vi "RT Main v0.91.vi"() -> ()   [LabVIEW 2017]
doc: "Changelog:\n\nv0.9:\n- Autocycle"
uses:
  Controls/Auto Delays.ctl
  support/Controls/All Inputs.ctl
  support/Controls/Index Details.ctl
  support/Controls/Auto Stats.ctl
  Controls/Auto Times.ctl
  Global Variables/RT GV.vi
  support/Message Queue/Enqueue Message (Single).vi
  Global Variables/FPGA GV.vi
  <vilib>/Utility/error.llb/Error Cluster From Error Code.vi
  <vilib>/rvi/errors/niLvFpgaAdjustHostInterfaceError.vi
  Global Variables/Network Globals.vi
  <vilib>/FPGAPlugInAG/Dynamic/niLvFpga_Close_Dynamic.vi
  <vilib>/rvi/interface/nirviReadWriteControl/nirviReadWriteControl.xnode
  Controls/FPGA Ref.ctl
  <vilib>/rvi/interface/nirviCloseFPGA/nirviCloseFPGA.xnode
  support/Message Queue/Message Queue.lvlib
  NiFpgaLv.dll
  <vilib>/rvi/interface/Simulation/niFpgaSimulationCallBeginRW.vi
panel:
  in  "Auto Para":T1={"Agitator Delays"=[700, 250], "TF Delays"=[700, 800, 2], "Insertion Delays"=[100, 500], "Cutting Delays"=[300, 300, 100], "PF Delays"=[250, 30000], "Measur. Delays"=[500.0, 188.9, 1.0], "Reject Delays"=[500], "BF Delays"=[1000, 1000]}
  in  "Counts in":cluster{"OutputCount":u32, "RejectCount":u32}
  in  "Stop Button 4":bool
  out "error out":errorcluster
  out "Wrong Message":string
  in  "Stop Button":bool
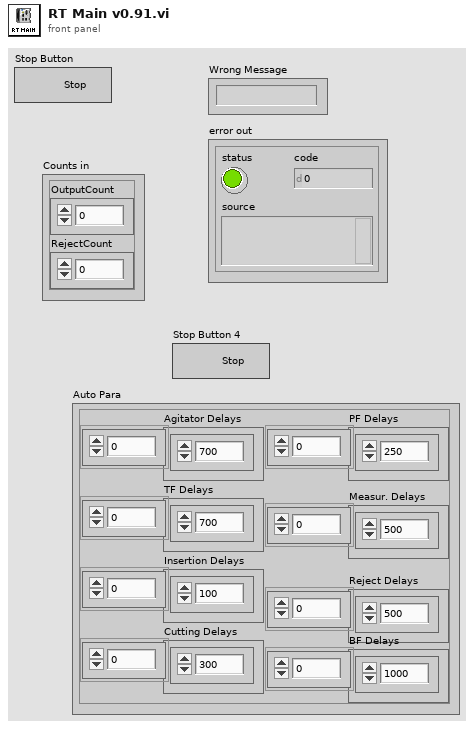
[diagram p1: front panel]
types:
  T1 = typedef "Auto Delays.ctl" = cluster{"Agitator Delays":u32[], "TF Delays":u32[], "Insertion Delays":u32[], "Cutting Delays":u32[], "PF Delays":u32[], "Measur. Delays":dbl[], "Reject Delays":u32[], "BF Delays":u32[]}
  T2 = typedef "FPGA Ref.ctl" = refnum<k20>
  T3 = cluster{"TL_Red":bool, "TL_Orange":bool, "TL_Green":bool, "TL_Buzzer":bool, "SOL_Index_Rotary_CW":bool, "SOL_Index_CNVR_Rotary_CCW":bool, "SOL_Index_CNVR_Stopper_Rear":bool, "SOL_Index_CNVR_Output _Separator _Rear":bool, "Bowl  Feeder_ ON":bool, "Pump_CNVR_Motor _ON":bool, "SOL_Gating_CYL_Rear":bool, "SOL_Tube_Feed_Agitatator":bool, "SOL_Tube_Feed_Gating_CYL":bool, "SOL_Insertion _CYL":bool, "SOL_Insertion_Clamp_CYL":bool, "SOL_Cutting_CYL":bool, "SOL_Cutting_Clamp_CYL":bool, "SOL_Insertion_Air_Nozzle":bool, "SOL_Measurement_CYL":bool, "SOL_Measure_Clamp_CYL":bool, "SOL_Rejection CYL_1":bool, "SOL_Rejection CYL_2":bool, "SOL_Rejection CYL_3":bool, "SOL_Rejection CYL_4":bool, "DO1.24":bool, "DO1.25":bool, "DO1.26":bool, "DO1.27":bool, "DO1.28":bool, "DO1.29":bool, "DO1.30":bool, "DO1.31":bool}
  T4 = typedef "All Inputs.ctl" = cluster{"DI 1":cluster{"Machine_ON":bool, "E_stop ":bool, "SW_Pressure":bool, "SW_Start ":bool, "SW_Reset":bool, "SW_Stop":bool, "SW_Door":bool, "RS_Index_Rotary_CW":bool, "RS_Index_Rotary_CCW":bool, "RS_Index_Stopper _Rear":bool, "RS_Index_Output_Separator_Rear":bool, "PES_Index_Pallet_Sensor":bool, "PES_Index_Output_Part Sensor":bool, "ICS_BF_Low_Level_1":bool, "ICS_BF_Low_Level_2":bool, "ICS_BF_Pump_CNVR_Full_1":bool, "ICS_BF_Pump_CNVR_Full_2":bool, "ICS_BF_Pump_CNVR_Full_3":bool, "ICS_BF_Pump_CNVR_Full_4":bool, "PES_PC_Pump Presence_1":bool, "PES_PC_Pump Presence_2":bool, "PES_PC_Pump Presence_3":bool, "PES_PC_Pump Presence_4":bool, "RS_PC_Gating_Front":bool, "PES_Pump_Interference":bool, "PES_TF_Low_Level":bool, "PES_Tube Presence_1":bool, "PES_Tube Presence_2":bool, "PES_Tube Presence_3":bool, "PES_Tube Presence_4":bool, "DI1.30":bool, "DI1.31":bool}, "DI 2":cluster{"RS_Agitatator_1_Rear ":bool, "RS_Agitatator_2_Rear ":bool, "RS_TF_Gating CYL_Rear":bool, "RS_Insertion_1_Rear":bool, "RS_Insertion_1_Front":bool, "RS_Insertion _2_Rear":bool, "RS_Insertion _2_Front":bool, "RS_Insertion _3_Rear":bool, "RS_Insertion _3_Front":bool, "RS_Insertion _4_Rear":bool, "RS_Insertion _4_Front":bool, "RS_Insertion_Clamp_Rear":bool, "RS_Cutting_Rear":bool, "RS_Cutting_Clamp _Rear":bool, "RS_Measurement_1_Rear":bool, "RS_Measurement_2_Rear":bool, "RS_Measurement_3_Rear":bool, "RS_Measurement_4_Rear":bool, "RS_Measure_Clamp_Rear":bool, "RS_Rejection_1_Rear":bool, "RS_Rejection_2_Rear":bool, "RS_Rejection_3_Rear":bool, "RS_Rejection_4_Rear":bool, "DI2.23":bool, "DI2.24":bool, "DI2.25":bool, "DI2.26":bool, "DI2.27":bool, "DI2.28":bool, "DI2.29":bool, "DI2.30":bool, "DI2.31":bool}, "IAS 1":dbl, "IAS 2":dbl, "IAS 3":dbl, "IAS 4":dbl, "DO 1":cluster{"TL_Red":bool, "TL_Orange":bool, "TL_Green":bool, "TL_Buzzer":bool, "SOL_Index_Rotary_CW":bool, "SOL_Index_CNVR_Rotary_CCW":bool, "SOL_Index_CNVR_Stopper_Rear":bool, "SOL_Index_CNVR_Output _Separator _Rear":bool, "Bowl  Feeder_ ON 1":bool, "Pump_CNVR_Motor _ON":bool, "SOL_PC_Gating_CYL_Rear":bool, "SOL_Tube_Feed_Agitatator":bool, "SOL_Tube_Feed_Gating_CYL":bool, "SOL_Insertion _CYL":bool, "SOL_Insertion_Clamp_CYL":bool, "SOL_Cutting_CYL":bool, "SOL_Cutting_Clamp_CYL":bool, "SOL_Insertion_Air_Nozzle":bool, "SOL_Measurement_CYL":bool, "DO1.19":bool, "SOL_Rejection CYL_1":bool, "SOL_Rejection CYL_2":bool, "SOL_Rejection CYL_3":bool, "SOL_Rejection CYL_4":bool, "Bowl  Feeder_ ON 2":bool, "SOL_BF_BlowerON":bool, "SOL_BF1_Track1":bool, "SOL_BF1_Track2":bool, "SOL_BF2_Track1":bool, "SOL_BF2_Track2":bool, "DO1.30":bool, "DO1.31":bool}}
  T5 = typedef "Index Details.ctl" = cluster{"Time (ms)":u32, "Waveform Graph":i16[]}
  T6 = cluster{T1, "Reject Pallets":cluster{"Reject 1":bool, "Reject 2":bool, "Reject 3":bool, "Reject 4":bool}}
  T7 = typedef "Auto Stats.ctl" = cluster{"Time":timestamp, "OEE":cluster{"AVL":dbl, "PRF":dbl, "QUA":dbl, "OEE":dbl}, "Auto Times":T8, "Counts out":cluster{"OutputCount":u32, "RejectCount":u32}, "Measurements":cluster{"1":dbl, "2":dbl, "3":dbl, "4":dbl}, "Outputs":cluster{"OutputCount":u32, "Numeric Control":u32}}
  T8 = typedef "Auto Times.ctl" = cluster{"Index Time":u32, "TF Time":u32, "Insertion Time":u32, "Cutting Time":u32, "PF Time":u32, "Meas. Time":u32, "Reject Time":u32}
  T9 = cluster{string, dbl, "Counts in":cluster{"OutputCount":u32, "RejectCount":u32}, "Auto Para":T1}
  T10 = cluster{"TL_Red":bool, "TL_Orange":bool, "TL_Green":bool, "TL_Buzzer":bool, "SOL_Index_Rotary_CW":bool, "SOL_Index_CNVR_Rotary_CCW":bool, "SOL_Index_CNVR_Stopper_Rear":bool, "SOL_Index_CNVR_Output _Separator _Rear":bool, "Bowl Feeder_ ON1":bool, "Pump_CNVR_Motor _ON":bool, "SOL_PC_Gating_CYL_Rear":bool, "SOL_Tube_Feed_Agitatator":bool, "SOL_Tube_Feed_Gating_CYL":bool, "SOL_Insertion _CYL":bool, "SOL_Insertion_Clamp_CYL":bool, "SOL_Cutting_CYL":bool, "SOL_Cutting_Clamp_CYL":bool, "SOL_Insertion_Air_Nozzle":bool, "SOL_Measurement_CYL":bool, "DO1.19":bool, "SOL_Rejection CYL_1":bool, "SOL_Rejection CYL_2":bool, "SOL_Rejection CYL_3":bool, "SOL_Rejection CYL_4":bool, "Bowl Feeder_ON2":bool, "SOL_BF_BlowerON":bool, "SOL_BF1_Track1":bool, "SOL_BF1_Track2":bool, "SOL_BF2_Track1":bool, "SOL_BF2_Track2":bool, "DO1.30":bool, "DO1.31":bool}
  T11 = cluster{"Machine_ON":bool, "E_stop ":bool, "SW_Pressure":bool, "SW_Start ":bool, "SW_Reset":bool, "SW_Stop":bool, "SW_Door":bool, "RS_Index_Rotary_CW":bool, "RS_Index_Rotary_CCW":bool, "RS_Index_Stopper _Rear":bool, "RS_Index_Output_Separator_Rear":bool, "PES_Index_Pallet_Sensor":bool, "PES_Index_Output_Part Sensor":bool, "ICS_BF_Low_Level_1":bool, "ICS_BF_Low_Level_2":bool, "ICS_BF_Pump_CNVR_Full_1":bool, "ICS_BF_Pump_CNVR_Full_2":bool, "ICS_BF_Pump_CNVR_Full_3":bool, "ICS_BF_Pump_CNVR_Full_4":bool, "PES_PC_Pump Presence_1":bool, "PES_PC_Pump Presence_2":bool, "PES_PC_Pump Presence_3":bool, "PES_PC_Pump Presence_4":bool, "RS_PC_Gating_Front":bool, "PES_Pump_Interference":bool, "PES_TF_Low_Level":bool, "PES_Tube Presence_1":bool, "PES_Tube Presence_2":bool, "PES_Tube Presence_3":bool, "PES_Tube Presence_4":bool, "DI1.30":bool, "DI1.31":bool}
  T12 = cluster{"RS_Agitatator_1_Rear ":bool, "RS_Agitatator_2_Rear ":bool, "RS_TF_Gating CYL_Rear":bool, "RS_Insertion_1_Rear":bool, "RS_Insertion_1_Front":bool, "RS_Insertion _2_Rear":bool, "RS_Insertion _2_Front":bool, "RS_Insertion _3_Rear":bool, "RS_Insertion _3_Front":bool, "RS_Insertion _4_Rear":bool, "RS_Insertion _4_Front":bool, "RS_Insertion_Clamp_Rear":bool, "RS_Cutting_Rear":bool, "RS_Cutting_Clamp _Rear":bool, "RS_Measurement_1_Rear":bool, "RS_Measurement_2_Rear":bool, "RS_Measurement_3_Rear":bool, "RS_Measurement_4_Rear":bool, "DI2.18":bool, "RS_Rejection_1_Rear":bool, "RS_Rejection_2_Rear":bool, "RS_Rejection_3_Rear":bool, "RS_Rejection_4_Rear":bool, "DI2.23":bool, "DI2.24":bool, "DI2.25":bool, "DI2.26":bool, "DI2.27":bool, "DI2.28":bool, "DI2.29":bool, "DI2.30":bool, "DI2.31":bool}
  T13 = cluster{"Array":string[][], "Machine Status":string}
  T14 = cluster{"Measurements":cluster{"1":dbl, "2":dbl, "3":dbl, "4":dbl}, "Reject Pallets":cluster{"Reject 1":bool, "Reject 2":bool, "Reject 3":bool, "Reject 4":bool}}
  T15 = cluster{"Auto Times":T8, "Results":cluster{"Measurements":cluster{"1":dbl, "2":dbl, "3":dbl, "4":dbl}, "Reject Pallets":cluster{"Reject 1":bool, "Reject 2":bool, "Reject 3":bool, "Reject 4":bool}}, "OutputCount":u32, "error out":errorcluster}
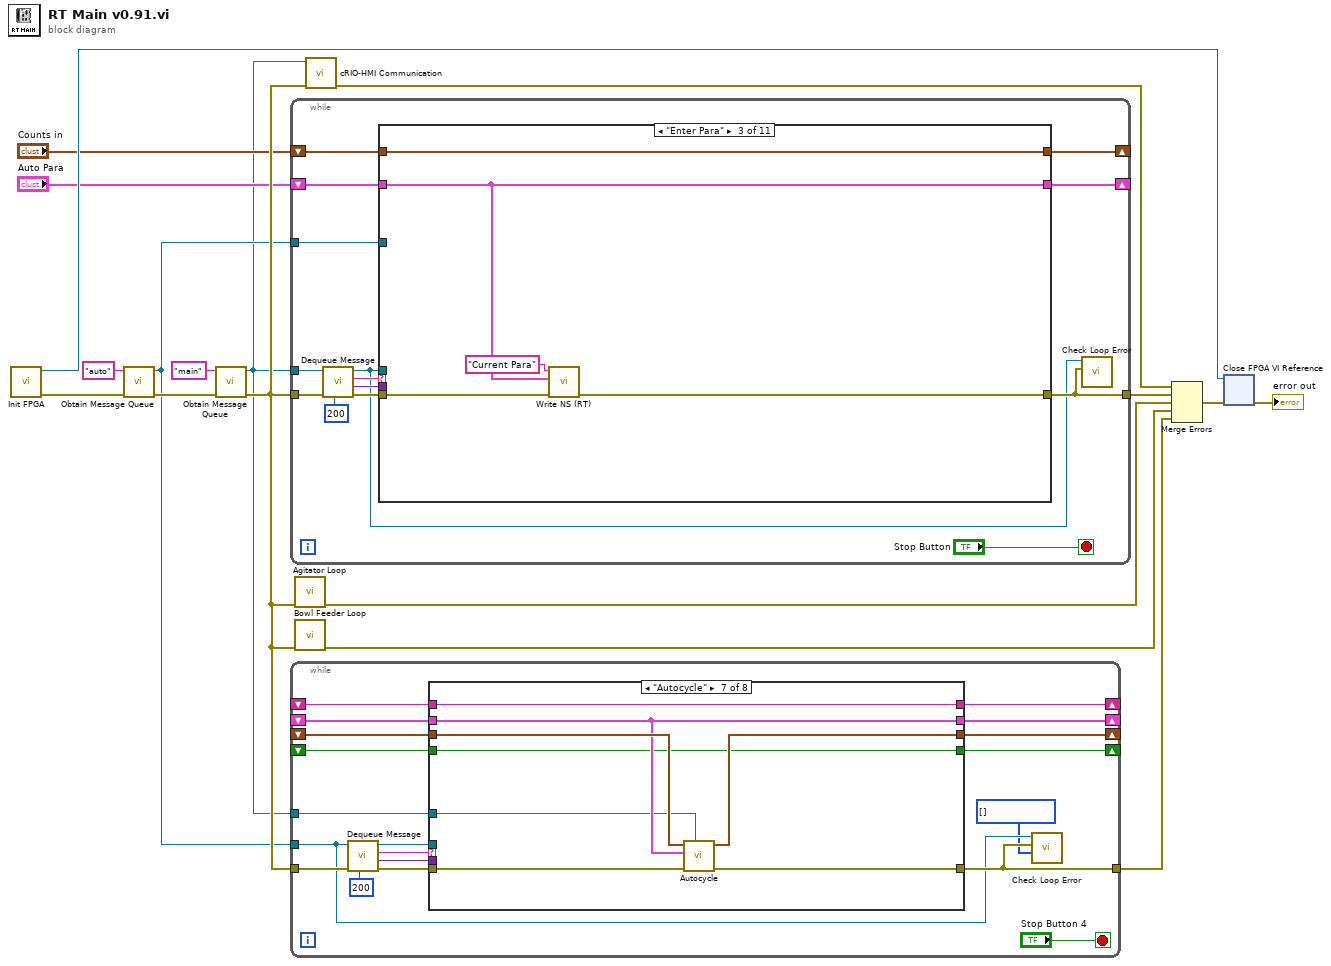
[diagram p0: block diagram]
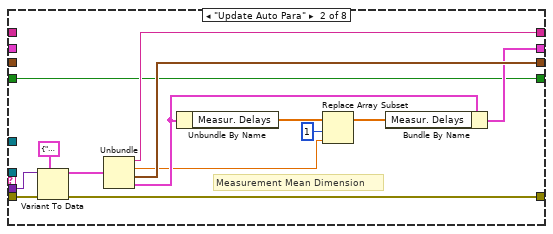
[diagram p3: hidden frame]
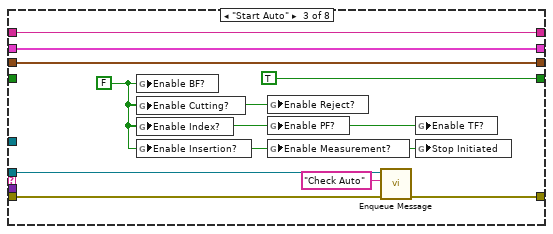
[diagram p4: hidden frame]
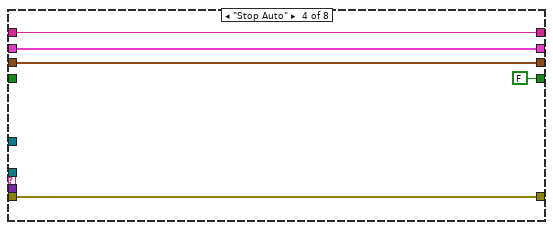
[diagram p5: hidden frame]
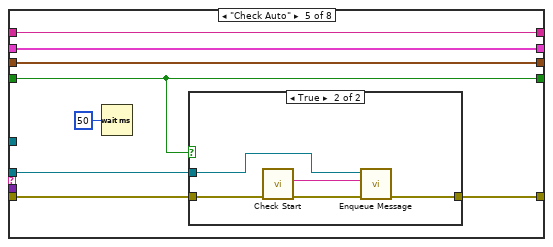
[diagram p6: hidden frame]
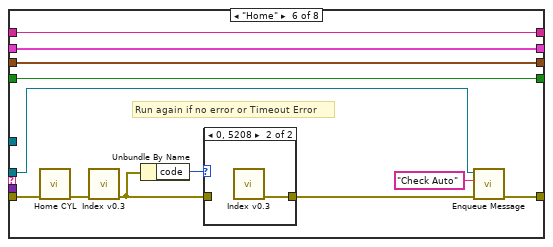
[diagram p8: hidden frame]
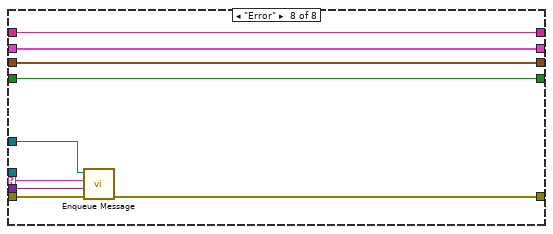
[diagram p10: hidden frame]
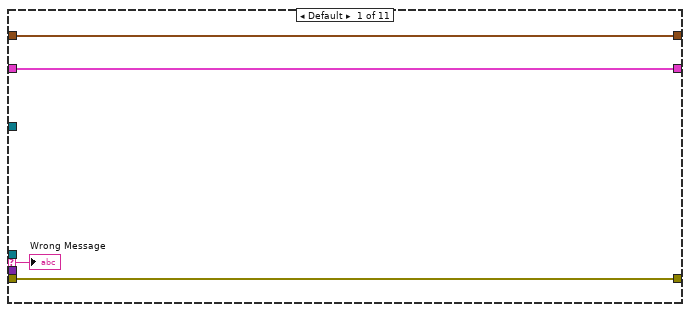
[diagram p11: hidden frame]
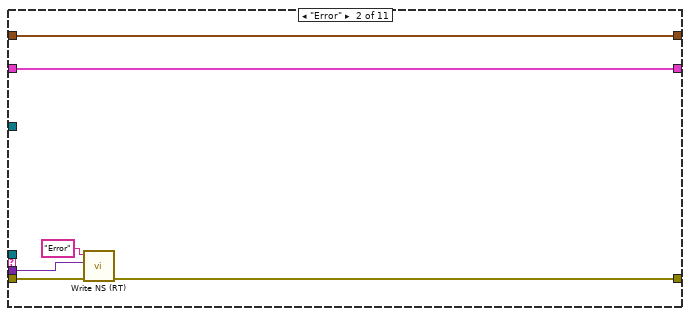
[diagram p12: hidden frame]
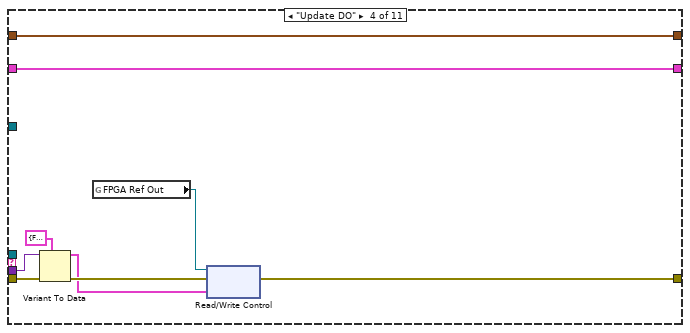
[diagram p13: hidden frame]
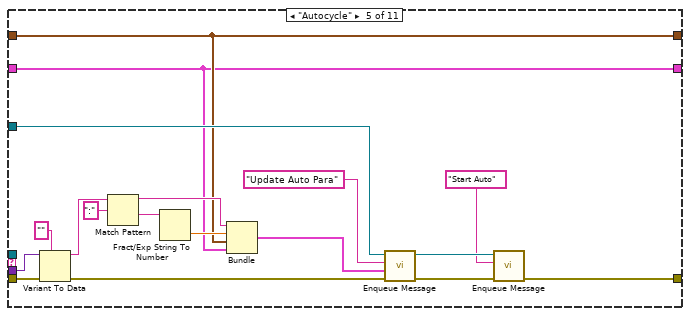
[diagram p14: hidden frame]
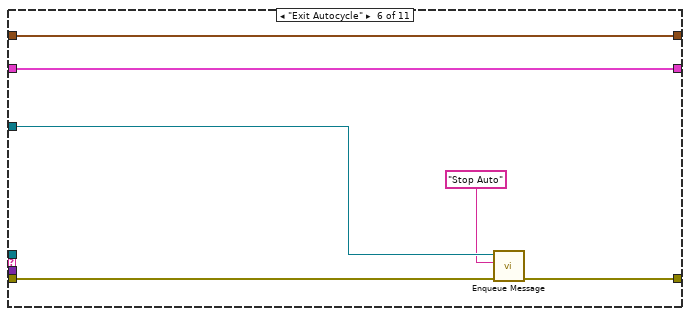
[diagram p15: hidden frame]
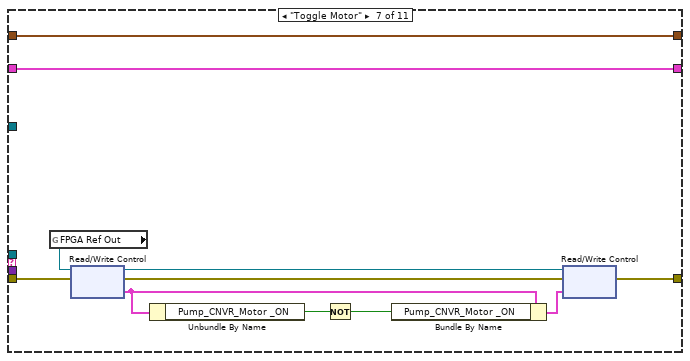
[diagram p16: hidden frame]
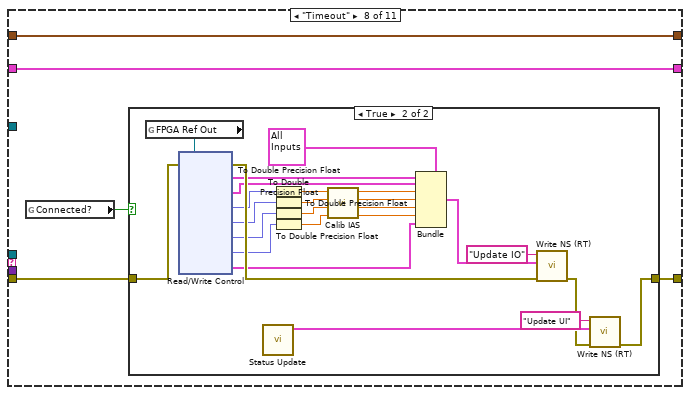
[diagram p17: hidden frame]
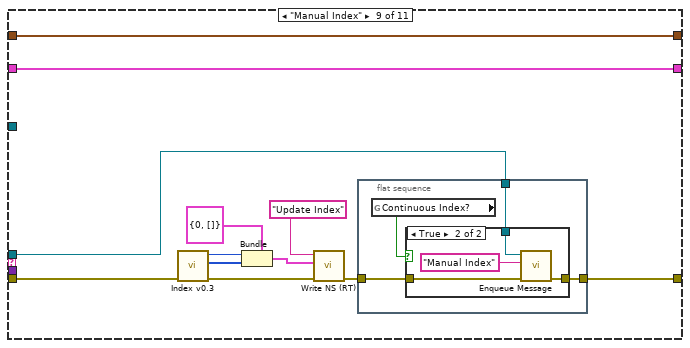
[diagram p19: hidden frame]
diagram:
  n1 = call "Init FPGA.vi"() -> ("error out"=w6:errorcluster, "FPGA Ref Out"=w11:T2)  [unwired: 10 in]
  n2 = call "Obtain Message Queue.vi"("error in (no error)"=w6, "name"="auto") -> ("error out"=w5:errorcluster, "Message Queue"=w2:refnum<queue>)  [unwired: 8 in]
  n3 = call "Obtain Message Queue.vi"("error in (no error)"=w5, "name"="main") -> ("error out"=w10:errorcluster, "Message Queue"=w1:refnum<queue>)  [unwired: 8 in]
  n4 = while {
    tunnel: w10 -> [w30]
    tunnel: w1 -> [w29]
    tunnel: [w25] -> w17
    tunnel: w2 -> [w22]
    shift-right: [w19] -> _
    shift-left: "Auto Para" -> [w20]
    shift-right: [w18] -> _
    shift-left: "Counts in" -> [w21]
    stop <- "Stop Button" stop-if-true
    n5 = call "Dequeue Message.vi"("timeout"=200, "error in (no error)"=w30, "Message Queue"=w29) -> ("error out"=w28:errorcluster, "Message Data"=w26:variant, "Message"=w27:string, "dup Message Queue"=w24:refnum<queue>)  [unwired: 5 in]
    n6 = case shown="\"Enter Para\"" w27 {
      selector: w27 -> [w35 _ _ _ _ _ _ _ _ _ _]
      tunnel: w28 -> [w34 w39 w46 w55 w73 w79 w89 w94 w133 w160 w170]
      tunnel: w24 -> [_ _ _ _ _ _ _ _ w125 _ _]
      tunnel: w26 -> [_ w37 _ w54 w72 _ _ _ _ w159 w169]
      tunnel: [w34 w38 w45 w50 w58 w75 w87 w95 w126 w155 w166] -> w25
      tunnel: w22 -> [_ _ _ _ w65 w78 _ _ _ _ _]
      tunnel: w21 -> [w33 w41 w43 w48 w62 w77 w81 w92 w122 w146 w165]
      tunnel: w20 -> [w32 w40 w42 w47 w61 w76 w80 w91 w123 w145 w164]
      tunnel: [w32 w40 w42 w47 w61 w76 w80 w91 w123 w145 w164] -> w19
      tunnel: [w33 w41 w43 w48 w62 w77 w81 w92 w122 w146 w165] -> w18
      frame Default {
        "Wrong Message" <- w35
      }
      frame "Error" {
        n7 = call "Write NS (RT).vi"("error in (no error)"=w39, "Message Data"=w37, "Message"="Error") -> ("error out"=w38:errorcluster)  [unwired: 8 in]
      }
      frame "Enter Para" {
        n8 = call "Write NS (RT).vi"("error in (no error)"=w46, "Message Data"=w42, "Message"="Current Para") -> ("error out"=w45:errorcluster)  [unwired: 8 in]
      }
      frame "Update DO" {
        n9 = Variant To Data(error in=w55, type=T3 {"TL_Red"=FALSE, "TL_Orange"=FALSE, "TL_Green"=FALSE, "TL_Buzzer"=FALSE, "SOL_Index_Rotary_CW"=FALSE, "SOL_Index_CNVR_Rotary_CCW"=FALSE, "SOL_Index_CNVR_Stopper_Rear"=FALSE, "SOL_Index_CNVR_Output _Separator _Rear"=FALSE, "Bowl  Feeder_ ON"=FALSE, "Pump_CNVR_Motor _ON"=FALSE, "SOL_Gating_CYL_Rear"=FALSE, "SOL_Tube_Feed_Agitatator"=FALSE, "SOL_Tube_Feed_Gating_CYL"=FALSE, "SOL_Insertion _CYL"=FALSE, "SOL_Insertion_Clamp_CYL"=FALSE, "SOL_Cutting_CYL"=FALSE, "SOL_Cutting_Clamp_CYL"=FALSE, "SOL_Insertion_Air_Nozzle"=FALSE, "SOL_Measurement_CYL"=FALSE, "SOL_Measure_Clamp_CYL"=FALSE, "SOL_Rejection CYL_1"=FALSE, "SOL_Rejection CYL_2"=FALSE, "SOL_Rejection CYL_3"=FALSE, "SOL_Rejection CYL_4"=FALSE, "DO1.24"=FALSE, "DO1.25"=FALSE, "DO1.26"=FALSE, "DO1.27"=FALSE, "DO1.28"=FALSE, "DO1.29"=FALSE, "DO1.30"=FALSE, "DO1.31"=FALSE} ("DO 1"), Variant=w54) -> (data=w49:T3, error out=w51:errorcluster)
        n10 = global read "FPGA GV.vi" "FPGA Ref Out"() -> (w52:T2)
        n11 = xnode "Read/Write Control"("FPGA VI Reference In"=w52, "error in"=w51, "DO 1"=w49) -> ("error out"=w50:errorcluster)  [unwired: 1 out]
      }
      frame "Autocycle" {
        n12 = Variant To Data(error in=w73, type="", Variant=w72) -> (data=w68:string, error out=w66:errorcluster)
        n13 = Match Pattern(string=w68, regular expression=":") -> (before substring=w64:string, after substring=w69:string)  [unwired: 1 in, 2 out]
        n14 = Fract/Exp String To Number(string=w69) -> (number=w63:dbl)  [unwired: 3 in, 1 out]
        n15 = Bundle(w64, w63, "Counts in"=w62, "Auto Para"=w61) -> (w60:T9)  [unwired: 1 in]
        n16 = call-poly "Enqueue Message.vi"("error in (no error)"=w66, "Message Data"=w60, "Message"="Update Auto Para", "Message Queue"=w65) -> ("error out"=w59:errorcluster, "dup Message Queue"=w57:refnum<queue>)  [unwired: 6 in]
        n17 = call-poly "Enqueue Message.vi"("error in (no error)"=w59, "Message"="Start Auto", "Message Queue"=w57) -> ("error out"=w58:errorcluster)  [unwired: 7 in, 1 out]
      }
      frame "Exit Autocycle" {
        n18 = call-poly "Enqueue Message.vi"("error in (no error)"=w79, "Message"="Stop Auto", "Message Queue"=w78) -> ("error out"=w75:errorcluster)  [unwired: 7 in, 1 out]
      }
      frame "Toggle Motor" {
        n19 = global read "FPGA GV.vi" "FPGA Ref Out"() -> (w90:T2)
        n20 = xnode "Read/Write Control"("FPGA VI Reference In"=w90, "error in"=w89) -> ("FPGA VI Reference Out"=w86:T2, "error out"=w88:errorcluster, "DO 1"=w84:T10)
        n21 = Unbundle By Name(w84) -> ("Pump_CNVR_Motor _ON"=w85:bool)
        n22 = Not(x=w85) -> (.not. x?=w82:bool)
        n23 = Bundle By Name(cluster=w84, "Pump_CNVR_Motor _ON"=w82) -> (w83:T10)
        n24 = xnode "Read/Write Control"("FPGA VI Reference In"=w86, "error in"=w88, "DO 1"=w83) -> ("error out"=w87:errorcluster)  [unwired: 1 out]
      }
      frame "Timeout" {
        n25 = global read "Network Globals.vi" "Connected?"() -> (w93:bool)
        n26 = case shown="True" w93 {
          tunnel: [w96 w98] -> w95
          tunnel: w94 -> [w96 w120]
          frame False {
          }
          frame True {
            n27 = global read "FPGA GV.vi" "FPGA Ref Out"() -> (w97:T2)
            n28 = xnode "Read/Write Control"("FPGA VI Reference In"=w97, "error in"=w120) -> ("error out"=w119:errorcluster, "DI 1"=w118:T11, "DI 2"=w117:T12, "AI0"=w116:fxp<+/-,27,6>, "AI1"=w115:fxp<+/-,27,6>, "AI2"=w114:fxp<+/-,27,6>, "AI3"=w113:fxp<+/-,27,6>, "DO 1"=w110:T10)  [unwired: 1 out]
            n29 = call "Status Update.vi"() -> ("Status Cluster"=w100:T13)  [unwired: 11 in]
            n30 = To Double Precision Float(number=w116) -> (double precision float=w103:dbl)
            n31 = To Double Precision Float(number=w115) -> (double precision float=w105:dbl)
            n32 = To Double Precision Float(number=w114) -> (double precision float=w107:dbl)
            n33 = To Double Precision Float(number=w113) -> (double precision float=w109:dbl)
            n34 = call "Calib IAS.vi"("x 4"=w109, "x 3"=w107, "x 2"=w105, "x"=w103) -> ("y 4"=w108:dbl, "y 3"=w106:dbl, "y 2"=w104:dbl, "y 1"=w102:dbl)  [unwired: 4 in]
            n35 = Bundle(cluster=T4 {"DI 1"={"Machine_ON"=FALSE, "E_stop "=FALSE, "SW_Pressure"=FALSE, "SW_Start "=FALSE, "SW_Reset"=FALSE, "SW_Stop"=FALSE, "SW_Door"=FALSE, "RS_Index_Rotary_CW"=FALSE, "RS_Index_Rotary_CCW"=FALSE, "RS_Index_Stopper _Rear"=FALSE, "RS_Index_Output_Separator_Rear"=FALSE, "PES_Index_Pallet_Sensor"=FALSE, "PES_Index_Output_Part Sensor"=FALSE, "ICS_BF_Low_Level_1"=FALSE, "ICS_BF_Low_Level_2"=FALSE, "ICS_BF_Pump_CNVR_Full_1"=FALSE, "ICS_BF_Pump_CNVR_Full_2"=FALSE, "ICS_BF_Pump_CNVR_Full_3"=FALSE, "ICS_BF_Pump_CNVR_Full_4"=FALSE, "PES_PC_Pump Presence_1"=FALSE, "PES_PC_Pump Presence_2"=FALSE, "PES_PC_Pump Presence_3"=FALSE, "PES_PC_Pump Presence_4"=FALSE, "RS_PC_Gating_Front"=FALSE, "PES_Pump_Interference"=FALSE, "PES_TF_Low_Level"=FALSE, "PES_Tube Presence_1"=FALSE, "PES_Tube Presence_2"=FALSE, "PES_Tube Presence_3"=FALSE, "PES_Tube Presence_4"=FALSE, "DI1.30"=FALSE, "DI1.31"=FALSE}, "DI 2"={"RS_Agitatator_1_Rear "=FALSE, "RS_Agitatator_2_Rear "=FALSE, "RS_TF_Gating CYL_Rear"=FALSE, "RS_Insertion_1_Rear"=FALSE, "RS_Insertion_1_Front"=FALSE, "RS_Insertion _2_Rear"=FALSE, "RS_Insertion _2_Front"=FALSE, "RS_Insertion _3_Rear"=FALSE, "RS_Insertion _3_Front"=FALSE, "RS_Insertion _4_Rear"=FALSE, "RS_Insertion _4_Front"=FALSE, "RS_Insertion_Clamp_Rear"=FALSE, "RS_Cutting_Rear"=FALSE, "RS_Cutting_Clamp _Rear"=FALSE, "RS_Measurement_1_Rear"=FALSE, "RS_Measurement_2_Rear"=FALSE, "RS_Measurement_3_Rear"=FALSE, "RS_Measurement_4_Rear"=FALSE, "RS_Measure_Clamp_Rear"=FALSE, "RS_Rejection_1_Rear"=FALSE, "RS_Rejection_2_Rear"=FALSE, "RS_Rejection_3_Rear"=FALSE, "RS_Rejection_4_Rear"=FALSE, "DI2.23"=FALSE, "DI2.24"=FALSE, "DI2.25"=FALSE, "DI2.26"=FALSE, "DI2.27"=FALSE, "DI2.28"=FALSE, "DI2.29"=FALSE, "DI2.30"=FALSE, "DI2.31"=FALSE}, "IAS 1"=0.0, "IAS 2"=0.0, "IAS 3"=0.0, "IAS 4"=0.0, "DO 1"={"TL_Red"=FALSE, "TL_Orange"=FALSE, "TL_Green"=FALSE, "TL_Buzzer"=FALSE, "SOL_Index_Rotary_CW"=FALSE, "SOL_Index_CNVR_Rotary_CCW"=FALSE, "SOL_Index_CNVR_Stopper_Rear"=FALSE, "SOL_Index_CNVR_Output _Separator _Rear"=FALSE, "Bowl  Feeder_ ON 1"=FALSE, "Pump_CNVR_Motor _ON"=FALSE, "SOL_PC_Gating_CYL_Rear"=FALSE, "SOL_Tube_Feed_Agitatator"=FALSE, "SOL_Tube_Feed_Gating_CYL"=FALSE, "SOL_Insertion _CYL"=FALSE, "SOL_Insertion_Clamp_CYL"=FALSE, "SOL_Cutting_CYL"=FALSE, "SOL_Cutting_Clamp_CYL"=FALSE, "SOL_Insertion_Air_Nozzle"=FALSE, "SOL_Measurement_CYL"=FALSE, "DO1.19"=FALSE, "SOL_Rejection CYL_1"=FALSE, "SOL_Rejection CYL_2"=FALSE, "SOL_Rejection CYL_3"=FALSE, "SOL_Rejection CYL_4"=FALSE, "Bowl  Feeder_ ON 2"=FALSE, "SOL_BF_BlowerON"=FALSE, "SOL_BF1_Track1"=FALSE, "SOL_BF1_Track2"=FALSE, "SOL_BF2_Track1"=FALSE, "SOL_BF2_Track2"=FALSE, "DO1.30"=FALSE, "DO1.31"=FALSE}}, "DI 1"=w118, "DI 2"=w117, "IAS 1"=w102, "IAS 2"=w104, "IAS 3"=w106, "IAS 4"=w108, "DO 1"=w110) -> (w112:T4)
            n36 = call "Write NS (RT).vi"("error in (no error)"=w119, "Message Data"=w112, "Message"="Update IO") -> ("error out"=w99:errorcluster)  [unwired: 8 in]
            n37 = call "Write NS (RT).vi"("error in (no error)"=w99, "Message Data"=w100, "Message"="Update UI") -> ("error out"=w98:errorcluster)  [unwired: 8 in]
          }
        }
      }
      frame "Manual Index" {
        n38 = call "Index v0.3.vi"("error in (no error)"=w133) -> ("error out"=w131:errorcluster, "Waveform Graph"=w129:i16[], "Index Time"=w130:u32)  [unwired: 7 in, 1 out]
        n39 = Bundle(cluster=T5 {"Time (ms)"=0, "Waveform Graph"=[]}, "Time (ms)"=w130, "Waveform Graph"=w129) -> (w128:T5)
        n40 = call "Write NS (RT).vi"("error in (no error)"=w131, "Message Data"=w128, "Message"="Update Index") -> ("error out"=w127:errorcluster)  [unwired: 8 in]
        n41 = flat-sequence {
          tunnel: w127 -> [w137]
          tunnel: [w136] -> w126
          tunnel: w125 -> [w134]
          frame #0 {
            n42 = global read "RT GV.vi" "Continuous Index?"() -> (w135:bool)
            n43 = case shown="True" w135 {
              tunnel: w137 -> [w138 w142]
              tunnel: [w138 w141] -> w136
              tunnel: w134 -> [_ w139]
              frame False {
              }
              frame True {
                n44 = call-poly "Enqueue Message.vi"("error in (no error)"=w142, "Message"="Manual Index", "Message Queue"=w139) -> ("error out"=w141:errorcluster)  [unwired: 7 in, 1 out]
              }
            }
          }
        }
      }
      frame "Manual Run" {
        n45 = Variant To Data(error in=w160, type=T6 {{"Agitator Delays"=[1000], "TF Delays"=[1000], "Insertion Delays"=[1000], "Cutting Delays"=[1000], "PF Delays"=[1000], "Measur. Delays"=[1000.0], "Reject Delays"=[1000], "BF Delays"=[1000]}, "Reject Pallets"={"Reject 1"=FALSE, "Reject 2"=FALSE, "Reject 3"=FALSE, "Reject 4"=FALSE}}, Variant=w159) -> (data=w151:T6, error out=w158:errorcluster)
        n46 = Unbundle(w151) -> (w148:T1)  [unwired: 1 out]
        n47 = Unbundle By Name(w148) -> ("Agitator Delays"=w144:u32[], "BF Delays"=w143:u32[])
        n48 = call "Manual.vi"("error in"=w158, "Auto Delays"=w148) -> ("error out"=w150:errorcluster, "OutputCount"=w149:u32, "Results"=w147:T14, "Auto Times"=w154:T8)  [unwired: 6 in]
        n49 = global write "RT GV.vi" "Agitator Delays"(w144) -> ()
        n50 = global write "RT GV.vi" "BF Delays"(w143) -> ()
        n51 = Bundle("Auto Times"=w154, "Results"=w147, "OutputCount"=w149, "error out"=w150) -> (w153:T15)  [unwired: 1 in]
        n52 = call "Write NS (RT).vi"("Message Data"=w153, "Message"="Manual Status") -> ("error out"=w156:errorcluster)  [unwired: 9 in]
        n53 = Merge Errors(w156) -> (w155:errorcluster)
      }
      frame "Log Cycle" {
        n54 = Variant To Data(error in=w170, type=T7 {"Time"=timestamp(0 s since 1904-01-01), "OEE"={"AVL"=100.0, "PRF"=100.0, "QUA"=100.0, "OEE"=0.0}, "Auto Times"={"Index Time"=0, "TF Time"=0, "Insertion Time"=0, "Cutting Time"=0, "PF Time"=0, "Meas. Time"=0, "Reject Time"=0}, "Counts out"={"OutputCount"=0, "RejectCount"=0}, "Measurements"={"1"=0.0, "2"=0.0, "3"=0.0, "4"=0.0}, "Outputs"={"OutputCount"=0, "Numeric Control"=0}} ("Auto Stats"), Variant=w169) -> (data=w161:T7, error out=w162:errorcluster)
        n55 = call "Write NS (RT).vi"("error in (no error)"=w162, "Message Data"=w161, "Message"="Autocycle Log") -> ("error out"=w167:errorcluster)  [unwired: 8 in]
        n56 = Merge Errors(w167) -> (w166:errorcluster)
      }
    }
    n57 = call "Check Loop Error.vi"("error to process"=w25, "Message Queue"=w24) -> ()  [unwired: 8 in, 2 out]
  }
  n58 = while {
    tunnel: w10 -> [w185]
    tunnel: [w183] -> w9
    shift-right: [w187] -> _
    shift-left: _ -> [w188]
    tunnel: w2 -> [w175]
    shift-right: [w179] -> _
    shift-left: _ -> [w178]
    shift-right: [w177] -> _
    shift-left: _ -> [w176]
    shift-right: [w174] -> _
    shift-left: _ -> [w173]
    tunnel: w1 -> [w172]
    stop <- "Stop Button 4" stop-if-true
    n59 = call "Dequeue Message.vi"("timeout"=200, "error in (no error)"=w185, "Message Queue"=w175) -> ("error out"=w184:errorcluster, "Message Data"=w180:variant, "Message"=w181:string, "dup Message Queue"=w182:refnum<queue>)  [unwired: 5 in]
    n60 = case shown="\"Autocycle\"" w181 {
      selector: w181 -> [_ _ _ _ _ _ _ w263]
      tunnel: w184 -> [w194 w208 w213 w219 w225 w244 w258 w261]
      tunnel: [w194 w207 w212 w219 w227 w239 w257 w260] -> w183
      tunnel: w188 -> [w193 _ w217 w222 w230 w248 w256 w267]
      tunnel: [w193 w202 w217 w222 w230 w248 w255 w267] -> w187
      tunnel: w182 -> [_ _ w211 _ w226 w237 _ _]
      tunnel: w180 -> [_ w206 _ _ _ _ _ w262]
      tunnel: [w192 w203 w216 w221 w229 w247 w254 w266] -> w179
      tunnel: w178 -> [w192 _ w216 w221 w229 w247 w254 w266]
      tunnel: [w191 w196 w215 w220 w228 w246 w253 w265] -> w177
      tunnel: w176 -> [w191 _ w215 w220 w228 w246 w253 w265]
      tunnel: [w190 w195 TRUE FALSE w224 w245 w251 w264] -> w174
      tunnel: w173 -> [w190 w195 _ _ w224 w245 w251 w264]
      tunnel: w172 -> [_ _ _ _ _ _ w252 w259]
      frame Default {
      }
      frame "Update Auto Para" {
        # "Measurement Mean Dimension"
        n61 = Variant To Data(error in=w208, type=T9 {"", 0.0, "Counts in"={"OutputCount"=0, "RejectCount"=0}, "Auto Para"={"Agitator Delays"=[], "TF Delays"=[], "Insertion Delays"=[], "Cutting Delays"=[], "PF Delays"=[], "Measur. Delays"=[], "Reject Delays"=[], "BF Delays"=[]}} ("cluster"), Variant=w206) -> (data=w204:T9, error out=w207:errorcluster)
        n62 = Unbundle(w204) -> (w203:string, w198:dbl, "Counts in"=w202:cluster{"OutputCount":u32, "RejectCount":u32}, "Auto Para"=w201:T1)
        n63 = Unbundle By Name(w201) -> ("Measur. Delays"=w200:dbl[])
        n64 = Replace Array Subset(array=w200, new element=w198, index=1) -> (w197:dbl[])
        n65 = Bundle By Name(cluster=w201, "Measur. Delays"=w197) -> (w196:T1)
      }
      frame "Start Auto" {
        w209 = FALSE ("Enable BF?")
        n66 = global write "RT GV.vi" "Enable BF?"(w209) -> ()
        n67 = global write "RT GV.vi" "Enable Cutting?"(w209) -> ()
        n68 = global write "RT GV.vi" "Enable Index?"(w209) -> ()
        n69 = global write "RT GV.vi" "Enable Insertion?"(w209) -> ()
        n70 = global write "RT GV.vi" "Enable Reject?"(w209) -> ()
        n71 = global write "RT GV.vi" "Enable PF?"(w209) -> ()
        n72 = global write "RT GV.vi" "Enable Measurement?"(w209) -> ()
        n73 = call-poly "Enqueue Message.vi"("error in (no error)"=w213, "Message"="Check Auto", "Message Queue"=w211) -> ("error out"=w212:errorcluster)  [unwired: 7 in, 1 out]
        n74 = global write "RT GV.vi" "Enable TF?"(w209) -> ()
        n75 = global write "RT GV.vi" "Stop Initiated"(w209) -> ()
      }
      frame "Stop Auto" {
      }
      frame "Check Auto" {
        n76 = Wait (ms)(milliseconds to wait=u32 50) -> ()  [unwired: 1 out]
        n77 = case shown="True" w224 {
          tunnel: [w231 w236] -> w227
          tunnel: w226 -> [_ w232]
          tunnel: w225 -> [w231 w235]
          frame False {
          }
          frame True {
            n78 = call "Check Start.vi"("error in"=w235) -> ("error out"=w234:errorcluster, "Message"=w233:string)  [unwired: 9 in]
            n79 = call-poly "Enqueue Message.vi"("error in (no error)"=w234, "Message"=w233, "Message Queue"=w232) -> ("error out"=w236:errorcluster)  [unwired: 7 in, 1 out]
          }
        }
      }
      frame "Home" {
        # "Run again if no error or Timeout Error"
        n80 = call "Home CYL.vi"("error in"=w244) -> ("error out"=w243:errorcluster)  [unwired: 10 in]
        n81 = call "Index v0.3.vi"("error in (no error)"=w243) -> ("error out"=w241:errorcluster)  [unwired: 7 in, 3 out]
        n82 = Unbundle By Name(w241) -> ("code"=w242:i32)
        n83 = case shown="0, 5208" w242 {
          tunnel: [w249 w250] -> w238
          tunnel: w241 -> [w249 _]
          frame Default {
          }
          frame 0, 5208 {
            n84 = call "Index v0.3.vi"() -> ("error out"=w250:errorcluster)  [unwired: 8 in, 3 out]
          }
        }
        n85 = call-poly "Enqueue Message.vi"("error in (no error)"=w238, "Message"="Check Auto", "Message Queue"=w237) -> ("error out"=w239:errorcluster)  [unwired: 7 in, 1 out]
      }
      frame "Autocycle" {
        n86 = call "Autocycle.vi"("Message Queue"=w252, "error in"=w258, "Auto Para"=w253, "Counts in"=w256) -> ("error out"=w257:errorcluster, "Counts out"=w255:cluster{"OutputCount":u32, "RejectCount":u32})  [unwired: 6 in]
      }
      frame "Error" {
        n87 = call-poly "Enqueue Message.vi"("error in (no error)"=w261, "Message Data"=w262, "Message"=w263, "Message Queue"=w259) -> ("error out"=w260:errorcluster)  [unwired: 6 in, 1 out]
      }
    }
    n88 = call "Check Loop Error.vi"("Ignore Errors"=i32[] [], "error to process"=w183, "Message Queue"=w175) -> ()  [unwired: 7 in, 2 out]
  }
  n89 = call "Agitator Loop.vi"("error in (no error)"=w10) -> ("error out"=w13:errorcluster)  [unwired: 10 in]
  n90 = call "Bowl Feeder Loop.vi"("error in (no error)"=w10) -> ("error out"=w12:errorcluster)  [unwired: 10 in]
  n91 = call "cRIO-HMI Communication.vi"("error in (no error)"=w10, "Message Queue"=w1) -> ("error out"=w16:errorcluster)  [unwired: 9 in]
  n92 = Merge Errors(w16, w17, w13, w12, w9) -> (w15:errorcluster)
  n93 = xnode ("Close FPGA VI Reference")("FPGA VI Reference In"=w11, "error in"=w15) -> ("error out"=→"error out":errorcluster)
